vi "Phasor Explorer.vi"() -> ()   [LabVIEW 2019]
uses:
  Decay & Gates Options.ctl
  Phasor Explorer Phasor Plot Info.ctl
  SEPL Parameters.ctl
  Phasor Explorer Display Parameters.ctl
  Type of Series.ctl
  Phasor Explorer Phasor Parameters.ctl
  Phasor Calculation Type.ctl
  SEPL Type.ctl
  Phasor Explorer Decay Parameters.ctl
  IRF Model.ctl
  Phasor Explorer Gate Parameters.ctl
  Gate Type.ctl
  Type of User-defined Function.ctl
  Phasor Explorer Detector Parameters.ctl
  Phasor Explorer Q [Element].ctl
  Phasor Explorer Q [Event] List.ctl
  Phasor Explorer Internal Variables.ctl
  Graphs/XY Graph/XY Plot Data.ctl
  Graphs/XY Graph/XY Graph Plot Properties.ctl
  Graphs/XY Graph/XY Graph Event.ctl
  <vilib>/Utility/miscctls.llb/LVPoint32TypeDef.ctl
  <vilib>/Utility/miscctls.llb/LVPointDoubleTypeDef.ctl
  Graphs/Cursor Info.ctl
  SEPXP Globals.vi
  Phasor_Abort Parallel Computation.vi
  User-defined Gate.vi
  Graphs/Plot Editor/Plot Editor.lvlib
  Notebook/Notebook.lvlib
  Graphs/XY Graph/XY Graph Add-Ons.lvlib
  Rich Text Box/Rich Text Box.lvlib
  Variant/Variant to Data/Variant to Data.lvlib
panel:
  in  "Abort":bool
  in  "Message":string
  in  "Animated Busy Icon":bool=TRUE
  in  "Display Tabs":T1(tab)
  in  "Show UC Ticks":bool
  out "original tau_m":dbl[unit] format="%#_5g"
  out "original  tau_ph":dbl[unit] format="%#_5g"
  out "Phasor Graph TipStrip":string
  out "current tau_m":dbl[unit] format="%#_5g"
  out "current tau_ph":dbl[unit] format="%#_5g"
  out "tau_i":dbl[unit] format="%#_5g"
  out "Phasor Graph":cluster{"X Array":dbl[], "Y Array":dbl[]}[](graph)
  out "f(tau) Graph TipStrip":string
  out "Numerical Solution":T2 {"Solution 2" format="%#_5g"; "Solution 1" format="%#_5g"}
  out "Analytical Solutions":T2 caption="Analytical Solution" {"Solution 2" format="%#_5g"; "Solution 1" format="%#_5g"}
  in  "Use Cursor":bool caption="Use Pseudo Phasor Graph Cursor"
  in  "Linear Coefficients":cluster{"u":dbl, "v":dbl} {"v" format="%#_5g"; "u" format="%#_5g"}
  out "f(tau) Graph":cluster{"X Array":dbl[], "Y Array":dbl[]}[](graph)
  out "a(b) Graph TipStrip":string
  out "Max Tau":dbl[unit] format="%#_5g"
  out "Min Tau":dbl[unit] format="%#_5g"
  out "a(b) Graph":cluster{"X Array":dbl[], "Y Array":dbl[]}[](graph)=[{"X Array"=[0.0, 0.01, 0.02, 0.03, 0.04, 0.05, 0.060000000000000005, 0.07, 0.08, 0.09, 0.09999999999999999, 0.10999999999999999, 0.11999999999999998, 0.12999999999999998, 0.13999999999999999, 0.15, 0.16, 0.17, 0.18000000000000002, 0.19000000000000003, 0.20000000000000004, 0.21000000000000005, 0.22000000000000006, 0.23000000000000007, 0.24000000000000007, 0.25000000000000006, 0.26000000000000006, 0.2700000000000001, 0.2800000000000001, 0.2900000000000001, 0.3000000000000001, 0.3100000000000001, 0.3200000000000001, 0.3300000000000001, 0.34000000000000014, 0.35000000000000014, 0.36000000000000015, 0.37000000000000016, 0.38000000000000017, 0.3900000000000002, 0.4000000000000002, 0.4100000000000002, 0.4200000000000002, 0.4300000000000002, 0.4400000000000002, 0.45000000000000023, 0.46000000000000024, 0.47000000000000025, 0.48000000000000026, 0.49000000000000027, 0.5000000000000002, 0.5100000000000002, 0.5200000000000002, 0.5300000000000002, 0.5400000000000003, 0.5500000000000003, 0.5600000000000003, 0.5700000000000003, 0.5800000000000003, 0.5900000000000003, 0.6000000000000003, 0.6100000000000003, 0.6200000000000003, 0.6300000000000003, 0.6400000000000003, 0.6500000000000004, 0.6600000000000004, 0.6700000000000004, 0.6800000000000004, 0.6900000000000004, 0.7000000000000004, 0.7100000000000004, 0.7200000000000004, 0.7300000000000004, 0.7400000000000004, 0.7500000000000004, 0.7600000000000005, 0.7700000000000005, 0.7800000000000005, 0.7900000000000005, 0.8000000000000005, 0.8100000000000005, 0.8200000000000005, 0.8300000000000005, 0.8400000000000005, 0.8500000000000005, 0.8600000000000005, 0.8700000000000006, 0.8800000000000006, 0.8900000000000006, 0.9000000000000006, 0.9100000000000006, 0.9200000000000006, 0.9300000000000006, 0.9400000000000006, 0.9500000000000006, 0.9600000000000006, 0.9700000000000006, 0.9800000000000006, 0.9900000000000007, 1.0000000000000007], "Y Array"=[0.0, 0.01, 0.02, 0.03, 0.04, 0.05, 0.060000000000000005, 0.07, 0.08, 0.09, 0.09999999999999999, 0.10999999999999999, 0.11999999999999998, 0.12999999999999998, 0.13999999999999999, 0.15, 0.16, 0.17, 0.18000000000000002, 0.19000000000000003, 0.20000000000000004, 0.21000000000000005, 0.22000000000000006, 0.23000000000000007, 0.24000000000000007, 0.25000000000000006, 0.26000000000000006, 0.2700000000000001, 0.2800000000000001, 0.2900000000000001, 0.3000000000000001, 0.3100000000000001, 0.3200000000000001, 0.3300000000000001, 0.34000000000000014, 0.35000000000000014, 0.36000000000000015, 0.37000000000000016, 0.38000000000000017, 0.3900000000000002, 0.4000000000000002, 0.4100000000000002, 0.4200000000000002, 0.4300000000000002, 0.4400000000000002, 0.45000000000000023, 0.46000000000000024, 0.47000000000000025, 0.48000000000000026, 0.49000000000000027, 0.5000000000000002, 0.5100000000000002, 0.5200000000000002, 0.5300000000000002, 0.5400000000000003, 0.5500000000000003, 0.5600000000000003, 0.5700000000000003, 0.5800000000000003, 0.5900000000000003, 0.6000000000000003, 0.6100000000000003, 0.6200000000000003, 0.6300000000000003, 0.6400000000000003, 0.6500000000000004, 0.6600000000000004, 0.6700000000000004, 0.6800000000000004, 0.6900000000000004, 0.7000000000000004, 0.7100000000000004, 0.7200000000000004, 0.7300000000000004, 0.7400000000000004, 0.7500000000000004, 0.7600000000000005, 0.7700000000000005, 0.7800000000000005, 0.7900000000000005, 0.8000000000000005, 0.8100000000000005, 0.8200000000000005, 0.8300000000000005, 0.8400000000000005, 0.8500000000000005, 0.8600000000000005, 0.8700000000000006, 0.8800000000000006, 0.8900000000000006, 0.9000000000000006, 0.9100000000000006, 0.9200000000000006, 0.9300000000000006, 0.9400000000000006, 0.9500000000000006, 0.9600000000000006, 0.9700000000000006, 0.9800000000000006, 0.9900000000000007, 1.0000000000000007]}]
  in  "Compute Delta Tau":bool
  out "Pseudo-Phase Lifetime Graph TipStrip":string
  out "Pseudo-Phase Lifetime Graph":cluster{"X Array":dbl[], "Y Array":dbl[]}[](graph)=[{"X Array"=[0.0, 1.0, 2.0, 3.0, 4.0, 5.0, 6.0, 7.0, 8.0, 9.0, 10.0, 11.0, 12.0, 13.0, 14.0, 15.0, 16.0, 17.0, 18.0, 19.0, 20.0, 21.0, 22.0, 23.0, 24.0, 25.0, 26.0, 27.0, 28.0, 29.0, 30.0, 31.0, 32.0, 33.0, 34.0, 35.0, 36.0, 37.0, 38.0, 39.0, 40.0, 41.0, 42.0, 43.0, 44.0, 45.0, 46.0, 47.0, 48.0, 49.0, 50.0, 51.0, 52.0, 53.0, 54.0, 55.0, 56.0, 57.0, 58.0, 59.0, 60.0, 61.0, 62.0, 63.0, 64.0, 65.0, 66.0, 67.0, 68.0, 69.0, 70.0, 71.0, 72.0, 73.0, 74.0, 75.0, 76.0, 77.0, 78.0, 79.0, 80.0, 81.0, 82.0, 83.0, 84.0, 85.0, 86.0, 87.0, 88.0, 89.0, 90.0, 91.0, 92.0, 93.0, 94.0, 95.0, 96.0, 97.0, 98.0, 99.0, 100.0], "Y Array"=[0.0, 1.0, 2.0, 3.0, 4.0, 5.0, 6.0, 7.0, 8.0, 9.0, 10.0, 11.0, 12.0, 13.0, 14.0, 15.0, 16.0, 17.0, 18.0, 19.0, 20.0, 21.0, 22.0, 23.0, 24.0, 25.0, 26.0, 27.0, 28.0, 29.0, 30.0, 31.0, 32.0, 33.0, 34.0, 35.0, 36.0, 37.0, 38.0, 39.0, 40.0, 41.0, 42.0, 43.0, 44.0, 45.0, 46.0, 47.0, 48.0, 49.0, 50.0, 51.0, 52.0, 53.0, 54.0, 55.0, 56.0, 57.0, 58.0, 59.0, 60.0, 61.0, 62.0, 63.0, 64.0, 65.0, 66.0, 67.0, 68.0, 69.0, 70.0, 71.0, 72.0, 73.0, 74.0, 75.0, 76.0, 77.0, 78.0, 79.0, 80.0, 81.0, 82.0, 83.0, 84.0, 85.0, 86.0, 87.0, 88.0, 89.0, 90.0, 91.0, 92.0, 93.0, 94.0, 95.0, 96.0, 97.0, 98.0, 99.0, 100.0]}]
  out "Decay & Gates Graph TipStrip":string
  in  "Decay & Gates Options":T3
  out "Decay & Gates Graph":cluster{"X Array":dbl[], "Y Array":dbl[]}[](graph)
  in  "Version":enum32{"Version 1", "Version 2"}(radio)=enum."Version 2"
  out "Sum of Gates Graph TipStrip":string
  out "Sum of Gates Graph":cluster{"X Array":dbl[], "Y Array":dbl[]}[](graph)
  out "Phasor Graph Plots Metadata":T4[](array[typedef]) {"Phasor Explorer Parameters"."Detector Parameters"."Frames/Image" min=1; "Phasor Explorer Parameters"."Detector Parameters"."Multiplicity" min=0; "Phasor Explorer Parameters"."Detector Parameters"."Bits/Frame" min=1; "Phasor Explorer Parameters"."Detector Parameters"."Gates/Frame" min=1; "Phasor Explorer Parameters"."Gate Parameters"."# Steps" min=0.0; "Phasor Explorer Parameters"."Gate Parameters"."Tolerance" min=0.0; "Phasor Explorer Parameters"."Gate Parameters"."Top Slope" min=0.0; "Phasor Explorer Parameters"."Gate Parameters"."Edge Width" min=0.0; "Phasor Explorer Parameters"."Gate Parameters"."Gate Step" min=0.0; "Phasor Explorer Parameters"."Gate Parameters"."# Gates" min=0.0 step=1.0; "Phasor Explorer Parameters"."Gate Parameters"."Gate Width" min=0.0; "Phasor Explorer Parameters"."Decay & IRF Parameters"."Lifetime" min=0.0; "Phasor Explorer Parameters"."Decay & IRF Parameters"."IRF Period" min=0.0; "Phasor Explorer Parameters"."Phasor Parameters"."Square Gate Width" min=0.0; "Phasor Explorer Parameters"."Phasor Parameters"."# Gates" min=0.0; "Phasor Explorer Parameters"."Phasor Parameters"."Calibration Lifetime" min=0.0; "Phasor Explorer Parameters"."Phasor Parameters"."Harmonic Frequency" min=0.0; "Phasor Explorer Parameters"."Display Parameters"."Min tau" min=0.0; "Phasor Explorer Parameters"."Display Parameters"."Max tau" min=0.0; "Phasor Explorer Parameters"."Display Parameters"."# Points" min=1 step=1}
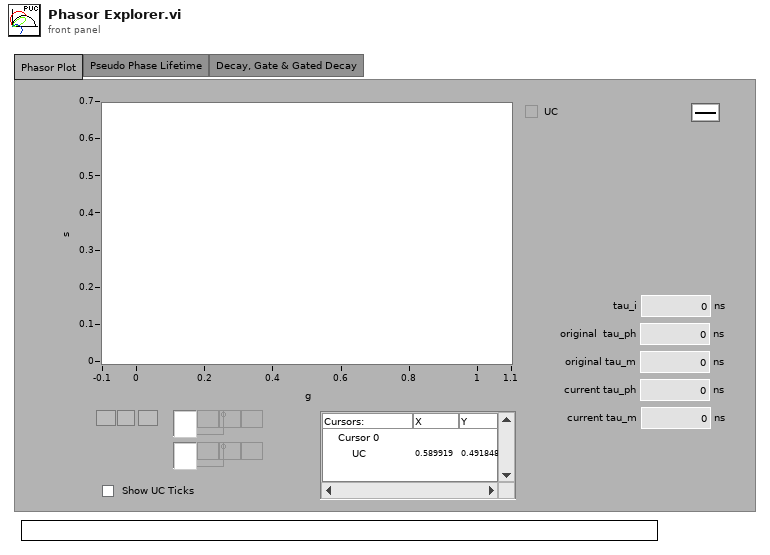
[diagram p1: front panel]
types:
  T1 = enum32{"Phasor Plot", "UC Intersections", "Alpha vs Beta", "Pseudo Phase Lifetime", "Decay, Gate & Gated Decay", "Sum of Gates", "Debug"}
  T2 = cluster{"Solution 1":dbl[unit], "Solution 2":dbl[unit]}
  T3 = typedef "Decay & Gates Options.ctl" = cluster{"Decay":bool, "Gate":bool, "Gated Decay":bool}
  T4 = typedef "Phasor Explorer Phasor Plot Info.ctl" = cluster{"Lifetime/Fraction Array":dbl[], "Phasor Explorer Parameters":T5, "Phase Lifetimes":dbl[], "Modulus Lifetimes":dbl[]}
  T5 = typedef "SEPL Parameters.ctl" = cluster{"Display Parameters":T6, "Phasor Parameters":T8, "Decay & IRF Parameters":T11, "Gate Parameters":T13, "Detector Parameters":T16}
  T6 = typedef "Phasor Explorer Display Parameters.ctl" = cluster{"# Points":i32, "Ramp Type":enum16{"Linear", "Logarithmic"}, "Type of Series":T7, "Min tau":dbl[unit], "Max tau":dbl[unit], "Include 0":bool, "Include Infinity":bool}
  T7 = typedef "Type of Series.ctl" = enum16{"1-Exp Decays", "Linear Combination of 1-Exp"}
  T8 = typedef "Phasor Explorer Phasor Parameters.ctl" = cluster{"Harmonic Frequency":dbl[unit], "Use f* = 1/D Frequency":bool, "Calibrated Phasor":bool, "Calibration Lifetime":dbl[unit], "Phasor Calculation":T9, "SEPL Type":T10, "# Gates":dbl, "Square Gate Width":dbl[unit], "Show Ticks":bool}
  T9 = typedef "Phasor Calculation Type.ctl" = enum16{"Direct Sum", "Analytical Formula"}
  T10 = typedef "SEPL Type.ctl" = enum16{"UC", "L_N", "L_N[W]", "L_X"}
  T11 = typedef "Phasor Explorer Decay Parameters.ctl" = cluster{"Lifetime":dbl[unit], "IRF Offset":dbl[unit], "IRF Period":dbl[unit], "Normalized Decays":bool, "IRF Model":T12, "IRF Parameter 1":dbl[unit]}
  T12 = typedef "IRF Model.ctl" = enum16{"Dirac", "Exponential"}
  T13 = typedef "Phasor Explorer Gate Parameters.ctl" = cluster{"First Gate Start":dbl[unit], "Use Gate Center":bool, "Gate Width":dbl[unit], "Gate Step":dbl[unit], "# Gates":dbl, "Gate Type":T14, "Edge Width":dbl[unit], "Top Slope":dbl[unit], "Reversed Sawtooth?":bool, "Analytical Computation":bool, "Integration":enum32{"Item 0", "Item 1"}, "Tolerance":dbl, "# Steps":dbl, "Type of User-defined Function":T15, "Use Gate Step":bool}
  T14 = typedef "Gate Type.ctl" = enum16{"Square", "Finite Edge Square", "Finite Edge, Tilted Top Square", "Triangle", "Sawtooth", "User-defined"}
  T15 = typedef "Type of User-defined Function.ctl" = enum16{"Gate", "IRF"}
  T16 = typedef "Phasor Explorer Detector Parameters.ctl" = cluster{"Frames/Image":i32, "Gates/Frame":i32, "Bits/Frame":i32, "Multiplicity":i32, "Incident Signal":dbl, "Poisson Signal":bool}
  T17 = typedef "Phasor Explorer Q [Event] List.ctl" = enum16{"Idle", "Initialization", "Show-Hide UC Ticks", "Edit User-defined Gate/IRF", "Update Phasor Graph", "Update Sum of Gates Graph", "Update Parameters", "Compute Decay &/or Gates", "Find Pseudo UC Intersections", "Compute alpha(beta) Plot", "Compute Pseudo-Phase Lifetime Plot", "Export Parameters to Clipboard", "Update Phase & Modulus Lifetime", "XY Graph Special Event", "Update Graph Plots Info", "Fit to Circle", "Quit"}
  T18 = enum32{"Phasor Plot", "UC Intersections", "Alpha vs Beta", "Pseudo Phase Lifetime", "Decay, Gate & Gated Decay", "Sum of Gates", "Debug"}[]
  T19 = typedef "Phasor Explorer Internal Variables.ctl" = cluster{"User-Defined Gate":T20, "User-defined Gate Plot Style":T21, "User-Defined IRF":T20}
  T20 = typedef "XY Plot Data.ctl" = cluster{"X Array":dbl[], "Y Array":dbl[]}
  T21 = typedef "XY Graph Plot Properties.ctl" = cluster{"Plot Index":i32, "Plot.Bar Plot Style":u8, "Plot.DigitalLineStyle":u8, "Plot.TransitionLocation":u8, "Plot.Transition Type":u8, "Plot.Fill To":i16, "Plot.Fill/Pt. Color":u32, "Plot.Label Format":u8, "Plot.Line Style":u8, "Plot.Line Width":u8, "Plot.Plot Color":u32, "Plot.Plot Interpolation":u8, "Plot.Plot Name":string, "Plot.Point Style":u8, "Plot.Visible?":bool, "Plot.XScaleIdx":u32, "Plot.YScaleIdx":u32, "Plot.Anti-aliased":bool}
  T22 = typedef "Phasor Explorer Q [Element].ctl" = cluster{"ZXP Q Event":T17, "Data":variant}
  T23 = typedef "Phasor Explorer Tipstrip Event Registration Refnums.ctl" = cluster{"Phasor Graph Event Registration Refnum":refnum<event-registration>, "Sum of Gates Graph Event Registration Refnum":refnum<event-registration>, "f(tau) Graph Event Registration Refnum":refnum<event-registration>, "a(b) Graph Event Registration Refnum":refnum<event-registration>, "Pseudo-Phase Lifetime Graph Event Registration Refnum":refnum<event-registration>, "Decay & Gate Graph Event Registration Refnum":refnum<event-registration>}
  T24 = enum32{"Phasor Plot", "UC Intersections", "Alpha vs Beta", "Pseudo Phase Lifetime", "Decay, Gate & Gated Decay", "Sum of Gates"}
  T25 = typedef "Cursor Info.ctl" = cluster{"CtlRef":refnum<vi>, "CursIdx":i32, "CursRef":refnum<vi>, "PlotIdx":i32, "PointIdx":i32, "CursLoc":cluster{"X":dbl, "Y":dbl}}
  T26 = typedef "XY Graph Add-Ons.lvlib/XY Graph Event.ctl" = cluster{"Item Tag":string, "XY Graph Refnum":refnum<vi>, "Coords":T27, "Item Path":string}
  T27 = typedef "LVPoint32TypeDef.ctl" = cluster{"Horizontal":i32, "Vertical":i32}
  T28 = typedef "LVPointDoubleTypeDef.ctl" = cluster{"X":dbl, "Y":dbl}
  T29 = cluster{"XY Graph Ref":refnum<vi>, "Mouse Coordinates":T28, "Plot Index":i32}
  T30 = typedef "Rich Text Box.lvlib/Text Formatting.ctl" = cluster{"Font":string, "Text Color":T31, "Text Background Color":T31, "Text Style":enum16{"Regular", "Bold", "Italic", "Underline", "Strikeout"}, "Font Size (Points)":dbl, "Text Alignment":i32}
  T31 = typedef "Rich Text Box.lvlib/Text Colors.ctl" = enum16{"Unchanged", "Black", "Blue", "Brown", "Gray", "Green", "Orange", "Pink", "Red", "White"}
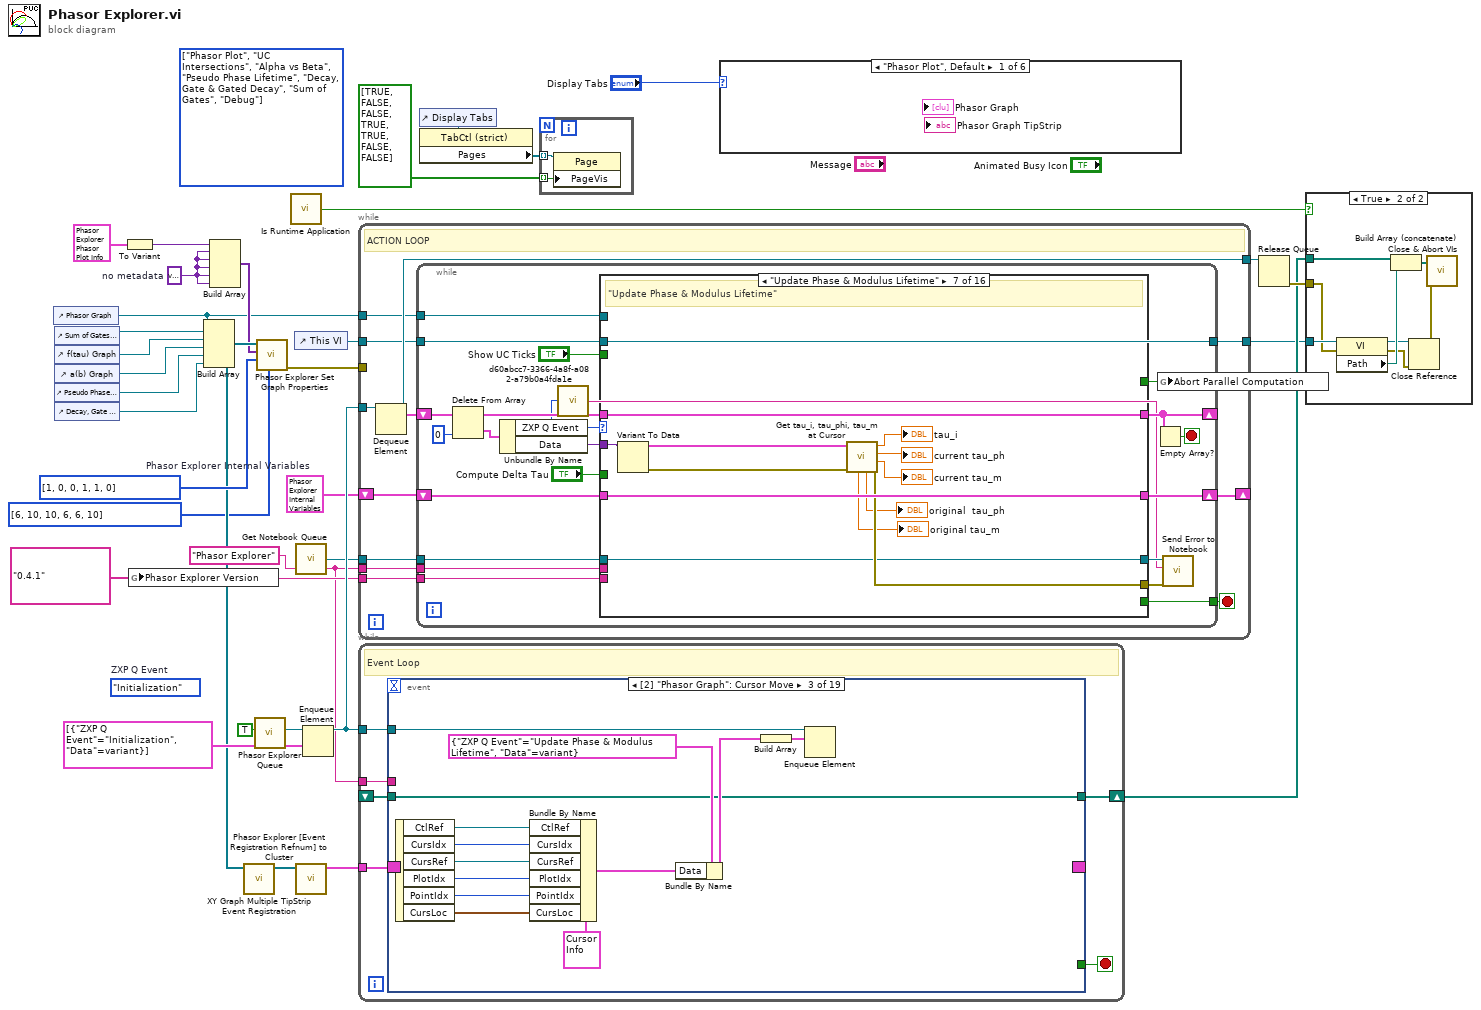
[diagram p0: block diagram]
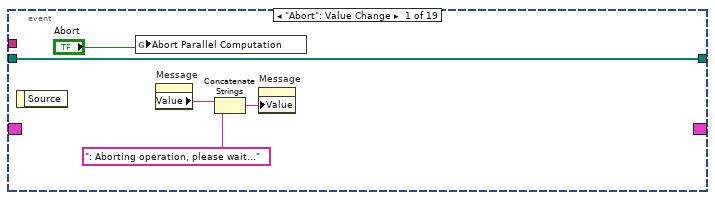
[diagram p3: hidden frame]
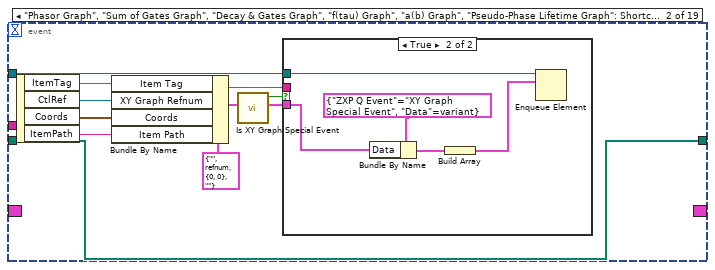
[diagram p4: hidden frame]
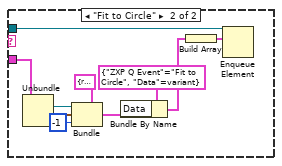
[diagram p6: hidden frame]
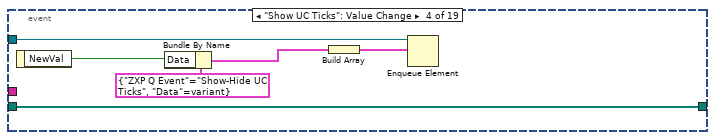
[diagram p7: hidden frame]
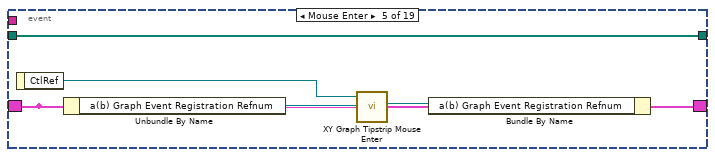
[diagram p8: hidden frame]
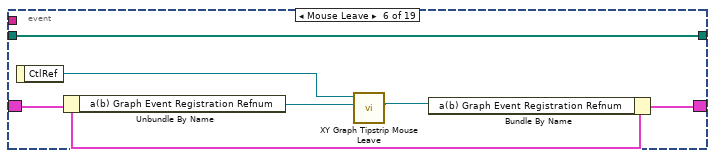
[diagram p9: hidden frame]
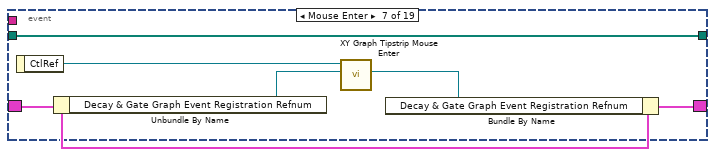
[diagram p10: hidden frame]
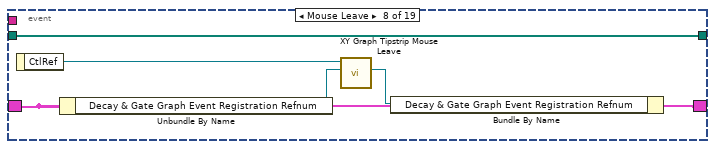
[diagram p11: hidden frame]
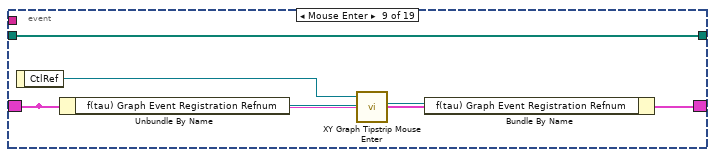
[diagram p12: hidden frame]
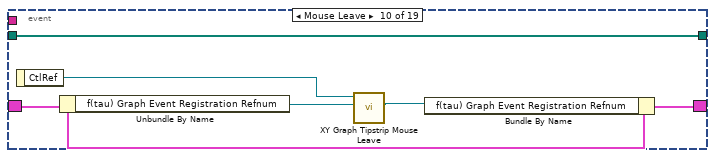
[diagram p13: hidden frame]
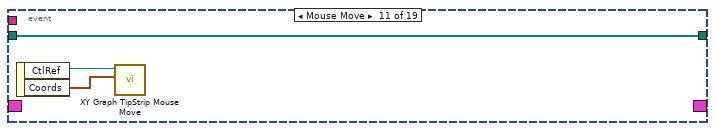
[diagram p14: hidden frame]
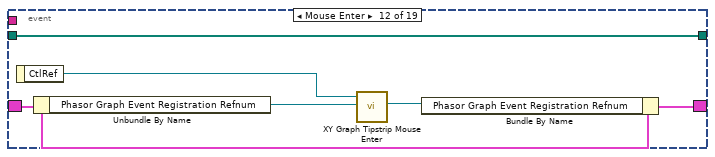
[diagram p15: hidden frame]
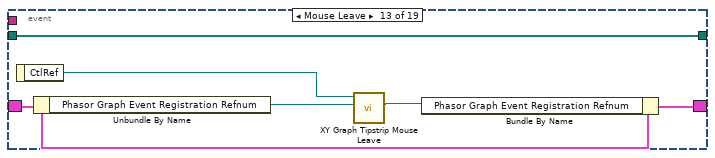
[diagram p16: hidden frame]
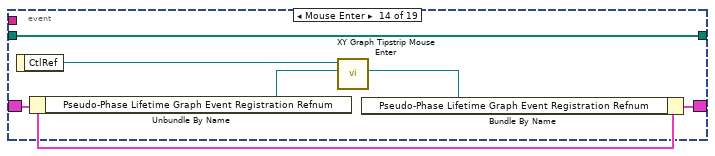
[diagram p17: hidden frame]
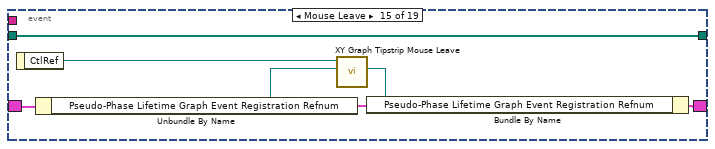
[diagram p18: hidden frame]
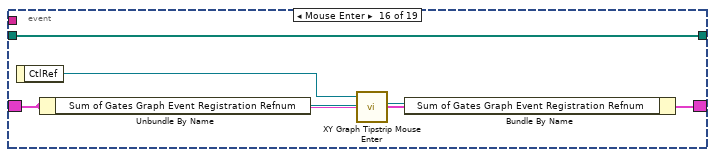
[diagram p19: hidden frame]
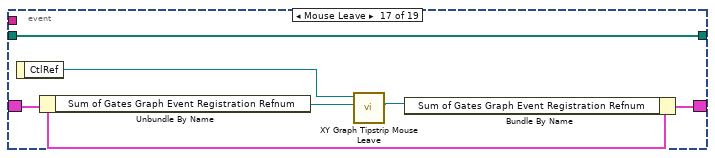
[diagram p20: hidden frame]
diagram:
  (unwired) Phasor_Explorer_Q_[Event]_List."Initialization"  # ZXP Q Event
  (unwired) T18 [enum."Phasor Plot", enum."UC Intersections", enum."Alpha vs Beta", enum."Pseudo Phase Lifetime", enum."Decay, Gate & Gated Decay", enum."Sum of Gates", enum."Debug"] items=["Phasor Plot", "UC Intersections", "Alpha vs Beta", "Pseudo Phase Lifetime", "Decay, Gate & Gated Decay", "Sum of Gates", "Debug"] ("Display Tabs")
  w9 = variant  # no metadata
  w15 = "Phasor Explorer" ("Phasor Explorer Version")
  w28 = "0.4.1" ("Phasor Explorer Version")
  w31 = T19 {"User-Defined Gate"={"X Array"=[], "Y Array"=[]}, "User-defined Gate Plot Style"={"Plot Index"=0, "Plot.Bar Plot Style"=0, "Plot.DigitalLineStyle"=0, "Plot.TransitionLocation"=0, "Plot.Transition Type"=0, "Plot.Fill To"=-1, "Plot.Fill/Pt. Color"=0, "Plot.Label Format"=0, "Plot.Line Style"=0, "Plot.Line Width"=0, "Plot.Plot Color"=0, "Plot.Plot Interpolation"=4, "Plot.Plot Name"="User-defined Gate", "Plot.Point Style"=0, "Plot.Visible?"=TRUE, "Plot.XScaleIdx"=0, "Plot.YScaleIdx"=0, "Plot.Anti-aliased"=TRUE}, "User-Defined IRF"={"X Array"=[], "Y Array"=[]}}  # Phasor Explorer Internal Variables
  n1 = control-ref of="Phasor Graph"() -> (w8:refnum<vi>)
  n2 = control-ref of="Sum of Gates Graph"() -> (w26:refnum<vi>)
  n3 = control-ref of="f(tau) Graph"() -> (w25:refnum<vi>)
  n4 = control-ref of="a(b) Graph"() -> (w24:refnum<vi>)
  n5 = control-ref of="Pseudo Phase Lifetime Graph"() -> (w23:refnum<vi>)
  n6 = control-ref of="Decay, Gate & Gated Decay Graph"() -> (w22:refnum<vi>)
  n7 = To Variant(anything=T4 {"Lifetime/Fraction Array"=[], "Phasor Explorer Parameters"={"Display Parameters"={"# Points"=0, "Ramp Type"=enum."Linear", "Type of Series"=enum."1-Exp Decays", "Min tau"=0.0, "Max tau"=0.0, "Include 0"=FALSE, "Include Infinity"=FALSE}, "Phasor Parameters"={"Harmonic Frequency"=0.0, "Use f* = 1/D Frequency"=FALSE, "Calibrated Phasor"=FALSE, "Calibration Lifetime"=1e-09, "Phasor Calculation"=enum."Direct Sum", "SEPL Type"=enum."UC", "# Gates"=1.0, "Square Gate Width"=1e-09, "Show Ticks"=FALSE}, "Decay & IRF Parameters"={"Lifetime"=0.0, "IRF Offset"=0.0, "IRF Period"=0.0, "Normalized Decays"=FALSE, "IRF Model"=enum."Dirac", "IRF Parameter 1"=0.0}, "Gate Parameters"={"First Gate Start"=0.0, "Use Gate Center"=FALSE, "Gate Width"=0.0, "Gate Step"=0.0, "# Gates"=0.0, "Gate Type"=enum."Square", "Edge Width"=0.0, "Top Slope"=0.0, "Reversed Sawtooth?"=FALSE, "Analytical Computation"=FALSE, "Integration"=enum."Item 0", "Tolerance"=1.0, "# Steps"=1.0, "Type of User-defined Function"=enum."Gate", "Use Gate Step"=FALSE}, "Detector Parameters"={"Frames/Image"=0, "Gates/Frame"=0, "Bits/Frame"=0, "Multiplicity"=0, "Incident Signal"=0.0, "Poisson Signal"=FALSE}}, "Phase Lifetimes"=[], "Modulus Lifetimes"=[]} ("Phasor Graph Plot Info")) -> (Variant=w11:variant)
  n8 = global write "SEPXP Globals.vi" "Phasor Explorer Version"(w28) -> ()
  n9 = Build Array(w8, w26, w25, w24, w23, w22) -> (w19:refnum<vi>[])
  n10 = Build Array(w11, w9, w9, w9, w9, w9) -> (w10:variant[])
  n11 = call "XY Graph Multiple TipStrip Event Registration.vi"("XY Graph Refnums"=w19) -> ("Tipstrips Event Registrations"=w18:refnum<event-registration>[])  [unwired: 9 in, 1 out]
  n12 = call "Phasor Explorer Queue.vi"("create if not found? (F)"=TRUE) -> ("Phasor Explorer Queue"=w14:refnum<queue>)  [unwired: 10 in]
  n13 = call "Phasor Explorer Set Graph Properties.vi"("Max Legend Size (8)"=i32[] [6, 10, 10, 6, 6, 10], "# Preserved PLots"=i32[] [1, 0, 0, 1, 1, 0], "Metadata Type"=w10, "XY Graph Ref Array"=w19) -> ("Error Out"=w21:errorcluster)  [unwired: 7 in]
  n14 = call "Is Runtime Application.vi"() -> ("Runtime ?"=w2:bool)  [unwired: 8 in, 1 out]
  n15 = control-ref of="This VI"() -> (w7:refnum<vi>)
  n16 = call "Get Notebook Queue.vi"() -> ("Notebook Queue"=w29:refnum<queue>)  [unwired: 9 in]
  n17 = call "Phasor Explorer [Event Registration Refnum] to Cluster.vi"("Tipstrips Event Registrations"=w18) -> ("Tipstrip RE refnums"=w17:T23)  [unwired: 10 in]
  n18 = Enqueue Element(queue=w14, element=T22[] [{"ZXP Q Event"=enum."Initialization", "Data"=variant}] ("PSEXP Q Element")) -> (queue out=w32:refnum<queue>)  [unwired: 2 in, 2 out]
  n19 = while {
    tunnel: w32 -> [w46]
    tunnel: [w44] -> w33
    tunnel: w7 -> [w42]
    shift-right: [w40] -> _
    shift-left: w31 -> [w41]
    tunnel: w29 -> [w39]
    tunnel: w28 -> [w38]
    tunnel: w15 -> [w37]
    tunnel: w21 -> [_]
    tunnel: w8 -> [w36]
    tunnel: [w35] -> w1
    stop <- w43 stop-if-true
    # "ACTION LOOP"
    n20 = Dequeue Element(queue=w46) -> (queue out=w44:refnum<queue>, element=w45:T22[])  [unwired: 2 in, 2 out]
    n21 = while {
      shift-right: [w64] -> _
      shift-left: w45 -> [w66]
      tunnel: [w62] -> w43
      tunnel: w42 -> [w48]
      shift-right: [w60] -> w40
      shift-left: w41 -> [w61]
      tunnel: w39 -> [w58]
      tunnel: w38 -> [w57]
      tunnel: w37 -> [w56]
      tunnel: w36 -> [w50]
      tunnel: [w48] -> w35
      stop <- w63 stop-if-true
      n22 = Delete From Array(array=w66, index=0) -> (deleted portion=w67:T22, array with subset deleted=w65:T22[])  [unwired: 1 in]
      n23 = Unbundle By Name(w67) -> ("ZXP Q Event"=w52:T17, "Data"=w59:variant)
      n24 = call "d60abcc7-3366-4a8f-a082-a79b0a4fda1e.vi"("Enum"=w52) -> ("String"=w51:string)
      n25 = case shown="\"Update Phase & Modulus Lifetime\"" w52 {
        tunnel: w65 -> [w71 w93 w122 w139 w160 w168 w180 w192 w201 w207 w217 w239 w248 w255 w266 _]
        tunnel: [w71 w93 w122 w139 w160 w168 w180 w192 w201 w207 w217 w239 w248 w255 w266 T22[] []] -> w64
        tunnel: [_ _ _ _ _ _ _ _ _ _ _ _ _ _ _ w271] -> w62
        tunnel: w48 -> [_ _ _ _ w157 w164 _ w183 w196 _ w211 w235 _ _ _ _]
        tunnel: w61 -> [w70 w77 w120 w126 w152 w165 w174 w189 w198 w204 w212 w236 w247 w254 w265 w275]
        tunnel: [w70 w77 w120 w127 w152 w165 w174 w189 w198 w204 w212 w236 w247 w254 w265 w275] -> w60
        tunnel: w59 -> [_ _ w109 w135 _ _ w179 _ _ _ _ _ w244 _ w264 _]
        tunnel: w58 -> [w69 w84 w121 w136 w153 w161 w172 w181 w193 w202 w208 w218 w240 w253 w261 w272]
        tunnel: w57 -> [_ w92 _ _ _ _ _ _ _ _ _ _ _ _ _ w274]
        tunnel: w56 -> [_ w91 _ _ _ _ _ _ _ _ _ _ _ _ _ w268]
        tunnel: "Compute Delta Tau" -> [_ _ _ _ _ _ _ _ w195 _ _ _ _ _ _ _]
        tunnel: [_ w86 w113 w137 w154 w162 w173 w182 w194 w203 w209 w219 w241 _ w259 w270] -> w54
        tunnel: [w69 w84 w121 w136 w153 w161 w172 w181 w193 w202 w208 w218 w240 w253 w261 w272] -> w53
        tunnel: w50 -> [_ w82 w115 _ _ _ _ _ _ _ _ _ _ w252 _ _]
        tunnel: [_ _ _ _ FALSE ("Abort") _ _ _ _ _ _ _ _ _ _ _] -> w47
        tunnel: "Show UC Ticks" -> [_ w72 _ _ _ _ _ _ _ _ _ _ _ _ _ _]
        frame "Idle", Default {
          # "\"Idle\", Default"
        }
        frame "Initialization" {
          # "\"Initialization\""
          n26 = call "Send Start-Stop Message.vi"("Start(T)/Stop(F)"=TRUE, "Version number"=w92, "Software Name"=w91, "Notebook Queue"=w84) -> ("Error Out"=w85:errorcluster)  [unwired: 7 in]
          n27 = call "Phasor Explorer Save-Load Settings.vi"("Load(F)/Save (T)"=FALSE) -> ("Error Out"=w89:errorcluster)  [unwired: 9 in, 1 out]
          n28 = call "9d87ee79-5232-47ce-8c93-ac6730099a75.vi"("# Steps (1)"=100) -> ("Ramp"=w101:dbl[])  [unwired: 8 in, 2 out]
          n29 = call "79f5c63b-0c71-4b9b-95d4-cbcc2b15c9cb.vi"("# Steps (1)"=100, "End (1)"=100.0) -> ("Ramp"=w106:dbl[])  [unwired: 7 in, 2 out]
          n30 = call "Get Harmonic Frequency.vi"("Error In"=w89) -> ("Error Out"=w75:errorcluster, "Harmonic frequency"=w76:dbl[unit])  [unwired: 2 in, 1 out]
          n31 = Bundle("Ramp"=w101, "Ramp"=w101) -> (w103:cluster{"Ramp":dbl[], "Ramp":dbl[]})  [unwired: 1 in]
          n32 = Bundle("Ramp"=w106, "Ramp"=w106) -> (w104:cluster{"Ramp":dbl[], "Ramp":dbl[]})  [unwired: 1 in]
          n33 = call "Universal Semicircle Plot.vi"("Error In"=w75, "Show Ticks"=w72, "Harmonic frequency"=w76) -> ("Error Out"=w74:errorcluster, "Universal Semi-circle"=w80:cluster{"X Array":dbl[], "Y Array":dbl[]})  [unwired: 6 in, 1 out]
          n34 = Build Array(w103) -> (w102:cluster{"Ramp":dbl[], "Ramp":dbl[]}[])
          n35 = Build Array(w104) -> (w105:cluster{"Ramp":dbl[], "Ramp":dbl[]}[])
          n36 = call "Phasor Explorer Update UC Lifetimes.vi"("Error In"=w74, "Harmonic Frequency"=w76, "Universal Semi-circle"=w80) -> ("Error Out"=w73:errorcluster, "PhXP UC Plot Info out"=w81:T4)  [unwired: 7 in]
          n37 = property on="a(b) Graph" class="XYGraph (strict)"("Value"=w102, "Active Plot"=u32 0, "Plot.Plot Name"="alpha = beta") -> ()  [unwired: 2 in, 2 out]
          n38 = property on="Pseudo-Phase Lifetime Graph" class="XYGraph (strict)"("Value"=w105, "Active Plot"=u32 0, "Plot.Plot Name"="tau = P-tau_ph") -> ()  [unwired: 2 in, 2 out]
          n39 = call "XY Graph Add Single Plot with Name.vi"("XYGraph Ref in"=w82, "Keep Existing Plots (T)"=FALSE, "Plot"=w80, "Plot Metadata"=w81, "Plot Name (\"Plot\")"="UC" ("Plot.Plot Name"), "error in (no error)"=w73) -> ("error out"=w78:errorcluster)  [unwired: 6 in, 3 out]
          n40 = Merge Errors(w78, w85) -> (w86:errorcluster)
          n41 = local write "Display Tabs"(T24."Phasor Plot" ("Display Tabs")) -> ()
        }
        frame "Show-Hide UC Ticks" {
          w112 = 0 ("Plot Idx")
          # "\"Show-Hide UC Ticks\""
          n42 = call "Variant to Boolean.vi"("Variant"=w109) -> ("Value"=w108:bool)  [unwired: 8 in]
          n43 = call "Get Harmonic Frequency.vi"() -> ("Error Out"=w119:errorcluster, "Harmonic frequency"=w118:dbl[unit])  [unwired: 3 in, 1 out]
          n44 = call "Universal Semicircle Plot.vi"("Tick Length"=0.02, "Error In"=w119, "Show Ticks"=w108, "Harmonic frequency"=w118) -> ("Error Out"=w117:errorcluster, "Universal Semi-circle"=w110:cluster{"X Array":dbl[], "Y Array":dbl[]})  [unwired: 5 in, 1 out]
          n45 = call "Phasor Explorer Update UC Lifetimes.vi"("Error In"=w117, "Harmonic Frequency"=w118, "Universal Semi-circle"=w110) -> ("Error Out"=w116:errorcluster, "PhXP UC Plot Info out"=w111:T4)  [unwired: 7 in]
          n46 = call "XY Graph Update Plot.vi"("Error In"=w116, "Plot"=w110, "Plot Idx"=w112, "XY Graph refnum"=w115) -> ("Error Out"=w114:errorcluster)  [unwired: 7 in]
          n47 = call "XY Graph Set Plot Metdata.vi"("error in (no error)"=w114, "Plot Metadata"=w111, "Plot Index (-1: last)"=w112, "XYGraph Ref in"=w115) -> ("error out"=w113:errorcluster)  [unwired: 5 in, 2 out]
        }
        frame "Edit User-defined Gate/IRF" {
          w125 = Type_of_User-defined_Function."IRF" ("Type of User-defined Function")
          # "\"Edit User-defined Gate/IRF\""
          n48 = Unbundle By Name(w126) -> ("User-Defined IRF"=w130:T20, "User-Defined Gate"=w131:T20, "User-defined Gate Plot Style"=w138:T21)
          n49 = Variant To Data(type=w125, Variant=w135) -> (data=w124:T15)  [unwired: 1 in, 1 out]
          n50 = Equal?(x=w125, y=w124) -> (x = y?=w123:bool)
          n51 = Select(t=w130, s=w123, f=w131) -> (s? t:f=w129:T20)
          n52 = Format Into String(format string="User-Defined %s Plot" ("Original Graph Name"), w124) -> (resulting string=w133:string)  [unwired: 2 in, 1 out]
          n53 = call "Plot Editor.vi"("Original Graph Name"=w133, "Plot Style in"=w138, "Plot in"=w129) -> ("Error Out"=w137:errorcluster, "Plot Style out"=w128:T21, "Plot out"=w132:T20)  [unwired: 6 in]
          n54 = case shown="\"Gate\", Default" w124 {
            tunnel: w132 -> [w140 w144]
            tunnel: w128 -> [w143 w147]
            tunnel: [w142 w146] -> w127
            tunnel: w126 -> [w141 w145]
            frame "Gate", Default {
              n55 = Bundle By Name(cluster=w141, "User-Defined Gate"=w140, "User-defined Gate Plot Style"=w143) -> (w142:T19)
              n56 = global write "User-defined Gate.vi" "User-defined Gate"(w140) -> ()
            }
            frame "IRF" {
              n57 = Bundle By Name(cluster=w145, "User-Defined IRF"=w144, "User-defined Gate Plot Style"=w147) -> (w146:T19)
              n58 = global write "User-defined Gate.vi" "User-defined IRF"(w144) -> ()
            }
          }
        }
        frame "Update Phasor Graph" {
          # "\"Update Phasor Graph\""
          n59 = call "Show Animated Busy Icon with Message and Abort Button.vi"("Message"="Computing Phasor Graph...") -> ("Error Out"=w159:errorcluster)  [unwired: 18 in]
          n60 = call "Compute SEPL Wrapper.vi"("error in (no error)"=w159, "VI in"=w157) -> ("error out"=w158:errorcluster, "Notebook String"=w149:string, "Plot Name"=w150:string)  [unwired: 7 in]
          n61 = call "Hide Animated Busy Icon with Message and Abort Button.vi"("Error In"=w158) -> ("Error Out"=w151:errorcluster)  [unwired: 18 in]
          n62 = call "Send PhXP Phasor Plot Info to Notebook.vi"("Graph Type"="Phasor", "error in (no error)"=w151, "Phasor Plot Info String"=w149, "Plot Name"=w150, "Notebook Queue"=w153) -> ("Error Out"=w154:errorcluster)  [unwired: 6 in]
        }
        frame "Update Sum of Gates Graph" {
          # "\"Update Sum of Gates Graph\""
          n63 = call "Show Animated Busy Icon with Message and Abort Button.vi"("Message"="Computing Sum of Gates...", "Target VI reference"=w164) -> ("Error Out"=w167:errorcluster)  [unwired: 17 in]
          n64 = call "Compute Sum of Gates Plot Wrapper.vi"("error in (no error)"=w167, "VI in"=w164) -> ("error out"=w166:errorcluster)  [unwired: 9 in]
          n65 = call "Hide Animated Busy Icon with Message and Abort Button.vi"("Error In"=w166) -> ("Error Out"=w162:errorcluster)  [unwired: 18 in]
        }
        frame "Update Phase & Modulus Lifetime" {
          # "\"Update Phase & Modulus Lifetime\""
          n66 = Variant To Data(Variant=w179) -> (data=w169:T25, error out=w175:errorcluster)  [unwired: 2 in]
          n67 = call "Get tau_i, tau_phi, tau_m at Cursor.vi"("Error In"=w175, "Cursor Info"=w169) -> ("Error Out"=w173:errorcluster, "current tau_m"=→"current tau_m":dbl[unit], "current tau_ph"=→"current tau_ph":dbl[unit], "tau_i"=→"tau_i":dbl[unit], "original tau_ph"=→"original  tau_ph":dbl[unit], "original tau_m"=→"original tau_m":dbl[unit])  [unwired: 4 in]
        }
        frame "Compute Decay &/or Gates" {
          # "\"Compute Decay &/or Gates\""
          n68 = call "Show Animated Busy Icon with Message and Abort Button.vi"("Message"="Computing Decay/Gates...", "Target VI reference"=w183) -> ("Error Out"=w191:errorcluster)  [unwired: 17 in]
          n69 = call "Compute Decay & Time Gates Wrapper.vi"("error in (no error)"=w191, "VI in"=w183) -> ("error out"=w190:errorcluster, "Decay & Gates Plot String"=w187:string, "Added Plot Name(s)"=w184:string)  [unwired: 6 in, 1 out]
          n70 = call "Hide Animated Busy Icon with Message and Abort Button.vi"("Target VI reference"=w183, "Error In"=w190) -> ("Error Out"=w186:errorcluster)  [unwired: 17 in]
          n71 = call "Send PhXP Phasor Plot Info to Notebook.vi"("Graph Type"="Decay & Gates", "error in (no error)"=w186, "Phasor Plot Info String"=w187, "Plot Name"=w184, "Notebook Queue"=w181) -> ("Error Out"=w182:errorcluster)  [unwired: 6 in]
        }
        frame "Compute Pseudo-Phase Lifetime Plot" {
          # "\"Compute Pseudo-Phase Lifetime Plot\""
          n72 = call "Show Animated Busy Icon with Message and Abort Button.vi"("Message"="Computing Phase Lifetime Plot...", "Target VI reference"=w196) -> ("Error Out"=w200:errorcluster)  [unwired: 17 in]
          n73 = call "Compute Gated Phase Lifetime Plot Wrapper.vi"("Compute Delta Tau"=w195, "error in (no error)"=w200, "VI in"=w196) -> ("error out"=w199:errorcluster)  [unwired: 8 in]
          n74 = call "Hide Animated Busy Icon with Message and Abort Button.vi"("Target VI reference"=w196, "Error In"=w199) -> ("Error Out"=w194:errorcluster)  [unwired: 17 in]
        }
        frame "Export Parameters to Clipboard" {
          # "\"Export Parameters to Clipboard\""
          n75 = call "Show Animated Busy Icon.vi"() -> ("Error Out"=w206:errorcluster)  [unwired: 9 in]
          n76 = call "Export Parameters to Clipboard Wrapper.vi"("error in (no error)"=w206) -> ("error out"=w205:errorcluster)  [unwired: 10 in]
          n77 = call "Hide Animated Busy Icon.vi"("Error In"=w205) -> ("Error Out"=w203:errorcluster)  [unwired: 8 in]
        }
        frame "Compute alpha(beta) Plot" {
          # "\"Compute alpha(beta) Plot\""
          n78 = call "Show Animated Busy Icon with Message and Abort Button.vi"("Message"="Computing Alpha(beta) Plot...", "Target VI reference"=w211) -> ("Error Out"=w216:errorcluster)  [unwired: 17 in]
          n79 = call "Compute alpha(beta) Plot Wrapper.vi"("error in (no error)"=w216, "VI in"=w211) -> ("error out"=w215:errorcluster, "Max Tau"=→"Max Tau":dbl[unit], "Min Tau"=→"Min Tau":dbl[unit])  [unwired: 7 in]
          n80 = call "Hide Animated Busy Icon with Message and Abort Button.vi"("Error In"=w215) -> ("Error Out"=w209:errorcluster)  [unwired: 18 in]
        }
        frame "Find Pseudo UC Intersections" {
          # "\"Find Pseudo UC Intersections\""
          n81 = call "Show Animated Busy Icon with Message.vi"("Message"="Computing UC Intersections...", "Target VI reference"=w235) -> ("Error Out"=w238:errorcluster)  [unwired: 9 in]
          n82 = call "Compute f(tau) & Zeros Wrapper.vi"("VI in"=w235, "error in (no error)"=w238) -> ("Numerical Solution 1"=w223:dbl[unit], "Numerical Solution 2"=w222:dbl[unit], "Analytical Solution 1"=w220:dbl[unit], "Analytical Solution 2"=w232:dbl[unit], "error out"=w237:errorcluster)  [unwired: 9 in]
          n83 = Not A Number/Path/Refnum?(number/path/refnum=w232) -> (NaN/Path/Refnum?=w233:bool)
          n84 = Not A Number/Path/Refnum?(number/path/refnum=w220) -> (NaN/Path/Refnum?=w231:bool)
          n85 = Not(x=w233) -> (.not. x?=w229:bool)
          n86 = call "Show Animated Busy Icon with Message and Abort Button.vi"("Error In"=w237) -> ("Error Out"=w219:errorcluster)  [unwired: 18 in]
          n87 = Not(x=w231) -> (.not. x?=w230:bool)
          n88 = Or(x=w230, y=w229) -> (x .or. y?=w228:bool)
          n89 = Not A Number/Path/Refnum?(number/path/refnum=w222) -> (NaN/Path/Refnum?=w227:bool)
          n90 = property on="Analytical Solutions" class="Clust (strict)"("Visible"=w228) -> ()  [unwired: 2 in, 2 out]
          n91 = property on="Solution 2" class="DigNum (strict)"("Value"=w232, "Visible"=w229) -> ()  [unwired: 2 in, 2 out]
          n92 = Not A Number/Path/Refnum?(number/path/refnum=w223) -> (NaN/Path/Refnum?=w226:bool)
          n93 = property on="Solution 1" class="DigNum (strict)"("Value"=w220, "Visible"=w230) -> ()  [unwired: 2 in, 2 out]
          n94 = Not(x=w227) -> (.not. x?=w221:bool)
          n95 = Not(x=w226) -> (.not. x?=w225:bool)
          n96 = Or(x=w225, y=w221) -> (x .or. y?=w224:bool)
          n97 = property on="Solution 1" class="DigNum (strict)"("Value"=w223, "Visible"=w225) -> ()  [unwired: 2 in, 2 out]
          n98 = property on="Solution 2" class="DigNum (strict)"("Value"=w222, "Visible"=w221) -> ()  [unwired: 2 in, 2 out]
          n99 = property on="Numerical Solution" class="Clust (strict)"("Visible"=w224) -> ()  [unwired: 2 in, 2 out]
        }
        frame "XY Graph Special Event" {
          # "\"XY Graph Special Event\""
          n100 = Variant To Data(Variant=w244) -> (data=w245:T26, error out=w246:errorcluster)  [unwired: 2 in]
          n101 = call "XY Graph Special Event Handler Wrapper.vi"("Error In"=w246, "XY Graph Event"=w245) -> ("Error Out"=w242:errorcluster, "Message"=w243:string)  [unwired: 8 in]
          n102 = call "Send Message to Notebook.vi"("Notebook Queue"=w240, "Message"=w243, "Error In"=w242) -> ("Error Out"=w241:errorcluster)  [unwired: 16 in]
        }
        frame "Update Graph Plots Info" {
          # "\"Update Graph Plots Info\""
          n103 = call "XY Graph Get Plots Metadata.vi"("XYGraph Ref"=w252) -> ("Plots Metadata"=w251:variant[])  [unwired: 7 in, 3 out]
          n104 = Variant To Data(type=T4[] [] ("Array"), Variant=w251) -> (data=→"Phasor Graph Plots Metadata":T4[])  [unwired: 1 in, 1 out]
        }
        frame "Fit to Circle" {
          # "\"Fit to Circle\""
          n105 = Variant To Data(Variant=w264) -> (data=w263:T29, error out=w262:errorcluster)  [unwired: 2 in]
          n106 = call "Fit Plot to Circle.vi"("Full Circle Plot"=FALSE, "Error In"=w262, "Circle Fit Plot Information"=w263) -> ("Error Out"=w260:errorcluster, "Result String"=w258:string)  [unwired: 6 in, 1 out]
          n107 = call "Result Style.vi"() -> ("Default Text Formatting"=w257:T30)
          n108 = call "Send Message to Notebook.vi"("Notebook Queue"=w261, "Message"=w258, "Error In"=w260, "Text Formatting"=w257) -> ("Error Out"=w259:errorcluster)  [unwired: 15 in]
        }
        frame "Quit" {
          w271 = TRUE
          # "\"Quit\""
          n109 = call "Send Start-Stop Message.vi"("Start(T)/Stop(F)"=FALSE, "Version number"=w274, "Software Name"=w268, "Notebook Queue"=w272) -> ("Error Out"=w269:errorcluster)  [unwired: 7 in]
          n110 = call "Delete Notebook Backup on Quit.vi"("Error In"=w269, "Main VI Name"=w268) -> ("Error Out"=w267:errorcluster)  [unwired: 9 in]
          n111 = call "Phasor Explorer Save-Load Settings.vi"("Load(F)/Save (T)"=w271, "Error In"=w267) -> ("Error Out"=w270:errorcluster)  [unwired: 8 in, 1 out]
        }
      }
      n112 = Empty Array?(array=w64) -> (empty?=w63:bool)
      n113 = global write "Phasor_Abort Parallel Computation.vi" "Abort Parallel Computation"(w47) -> ()
      n114 = call "Send Error to Notebook.vi"("error in (no error)"=w54, "State Machine Case Error Source"=w51, "Notebook Q"=w53) -> ()  [unwired: 8 in, 1 out]
    }
  }
  n115 = while {
    tunnel: w32 -> [w282]
    tunnel: w17 -> [w280]
    tunnel: w15 -> [w279]
    shift-right: [w278] -> w6
    shift-left: _ -> [w277]
    stop <- w281 stop-if-true
    # "Event Loop"
    n116 = event shown="[2] \"Phasor Graph\": Cursor Move" {
      selector: w280 -> [_ _ _ _ w338 w346 w350 w358 w362 w370 _ w377 w385 w389 w397 w401 w409 _ _]
      dyn-events: [_ _ _ _ w336 w345 w348 w357 w360 w369 _ w375 w384 w387 w396 w399 w408 _ _] -> _
      timeout: _ -> [_ _ _ _ _ _ _ _ _ _ _ _ _ _ _ _ _ _ _]
      tunnel: [_ _ _ _ _ _ _ _ _ _ _ _ _ _ _ _ _ w414 w458] -> w281
      tunnel: w282 -> [_ w292 w328 w334 _ _ _ _ _ _ _ _ _ _ _ _ _ w410 w460]
      tunnel: w279 -> [_ _ _ _ _ _ _ _ _ _ _ _ _ _ _ _ _ w413 w459]
      tunnel: [w284 w290 w316 w329 w335 w341 w347 w353 w359 w365 w371 w374 w380 w386 w392 w398 w404 w412 w461] -> w278
      tunnel: w277 -> [w284 w290 w316 w329 w335 w341 w347 w353 w359 w365 w371 w374 w380 w386 w392 w398 w404 w411 w461]
      event "Abort": Value Change {
        n117 = event-data() -> ()  [unwired: 1 in, 1 out]
        n118 = global write "Phasor_Abort Parallel Computation.vi" "Abort Parallel Computation"("Abort") -> ()
        n119 = property on="Message" class="Str"() -> ("Value"=w287:string)  [unwired: 2 in, 2 out]
        n120 = Concatenate Strings(w287, ": Aborting operation, please wait..." ("string")) -> (w285:string)
        n121 = property on="Message" class="Str"("Value"=w285) -> ()  [unwired: 2 in, 2 out]
      }
      event "Phasor Graph", "Sum of Gates Graph", "Decay & Gates Graph", "f(tau) Graph", "a(b) Graph", "Pseudo-Phase Lifetime Graph": Shortcut Menu Selection (User) {
        n122 = event-data() -> ("ItemTag"=w291:string, "CtlRef"=w296:refnum<vi>, "Coords"=w295:T27, "ItemPath"=w289:string)  [unwired: 1 in]
        n123 = Bundle By Name(cluster=T26 {"Item Tag"="", "XY Graph Refnum"=refnum, "Coords"={"Horizontal"=0, "Vertical"=0}, "Item Path"=""} ("XY Graph Event"), "Item Tag"=w291, "XY Graph Refnum"=w296, "Coords"=w295, "Item Path"=w289) -> (w297:T26)
        n124 = call "Is XY Graph Special Event.vi"("XY Graph Event"=w297) -> ("XY Graph Event"=w293:T26, "Special Event"=w294:bool)  [unwired: 8 in, 1 out]
        n125 = case shown="True" w294 {
          tunnel: w293 -> [w298 w313]
          tunnel: w292 -> [w299 w315]
          tunnel: w291 -> [w300 _]
          frame False {
            n126 = case shown="\"\", Default" w300 {
              tunnel: w299 -> [_ w309]
              tunnel: w298 -> [_ w310]
              frame "", Default {
              }
              frame "Fit to Circle" {
                n127 = Unbundle(w310) -> ("XY Graph Refnum"=w305:refnum<vi>, "Coords"=w304:T27)  [unwired: 2 out]
                n128 = Bundle(cluster=T29 {"XY Graph Ref"=refnum, "Mouse Coordinates"={"X"=0.0, "Y"=0.0}, "Plot Index"=0} ("data"), "XY Graph Ref"=w305, "Mouse Coordinates"=w304, "Plot Index"=-1) -> (w303:T29)
                n129 = Bundle By Name(cluster=T22 {"ZXP Q Event"=enum."Fit to Circle", "Data"=variant} ("element"), "Data"=w303) -> (w307:T22)
                n130 = Build Array(w307) -> (w306:T22[])
                n131 = Enqueue Element(queue=w309, element=w306) -> ()  [unwired: 2 in, 3 out]
              }
            }
          }
          frame True {
            n132 = Bundle By Name(cluster=T22 {"ZXP Q Event"=enum."XY Graph Special Event", "Data"=variant} ("element"), "Data"=w313) -> (w312:T22)
            n133 = Build Array(w312) -> (w311:T22[])
            n134 = Enqueue Element(queue=w315, element=w311) -> ()  [unwired: 2 in, 3 out]
          }
        }
      }
      event "Phasor Graph": Cursor Move {
        n135 = event-data() -> ("CtlRef"=w318:refnum<vi>, "CursIdx"=w324:i32, "CursRef"=w319:refnum<vi>, "PlotIdx"=w323:i32, "PointIdx"=w322:i32, "CursLoc"=w321:cluster{"X":dbl, "Y":dbl})  [unwired: 1 in]
        n136 = Bundle By Name(cluster=T25 {"CtlRef"=refnum, "CursIdx"=0, "CursRef"=refnum, "PlotIdx"=0, "PointIdx"=0, "CursLoc"={"X"=0.0, "Y"=0.0}} ("output cluster"), "CtlRef"=w318, "CursIdx"=w324, "CursRef"=w319, "PlotIdx"=w323, "PointIdx"=w322, "CursLoc"=w321) -> (w320:T25)
        n137 = Bundle By Name(cluster=T22 {"ZXP Q Event"=enum."Update Phase & Modulus Lifetime", "Data"=variant} ("element"), "Data"=w320) -> (w326:T22)
        n138 = Build Array(w326) -> (w325:T22[])
        n139 = Enqueue Element(queue=w328, element=w325) -> ()  [unwired: 2 in, 3 out]
      }
      event "Show UC Ticks": Value Change {
        n140 = event-data() -> ("NewVal"=w332:bool)  [unwired: 1 in]
        n141 = Bundle By Name(cluster=T22 {"ZXP Q Event"=enum."Show-Hide UC Ticks", "Data"=variant} ("element"), "Data"=w332) -> (w331:T22)
        n142 = Build Array(w331) -> (w330:T22[])
        n143 = Enqueue Element(queue=w334, element=w330) -> ()  [unwired: 2 in, 3 out]
      }
      event Mouse Enter {
        n144 = event-data() -> ("CtlRef"=w339:refnum<vi>)  [unwired: 1 in]
        n145 = Unbundle By Name(w338) -> ("a(b) Graph Event Registration Refnum"=w340:refnum<event-registration>)
        n146 = call "XY Graph Tipstrip Mouse Enter.vi"("Event Registration Refnum"=w340, "XY Graph Refnum"=w339) -> ("Event Registration Refnum"=w337:refnum<event-registration>)  [unwired: 8 in, 1 out]
        n147 = Bundle By Name(cluster=w338, "a(b) Graph Event Registration Refnum"=w337) -> (w336:T23)
      }
      event Mouse Leave {
        n148 = event-data() -> ("CtlRef"=w342:refnum<vi>)  [unwired: 1 in]
        n149 = Unbundle By Name(w346) -> ("a(b) Graph Event Registration Refnum"=w344:refnum<event-registration>)
        n150 = call "XY Graph Tipstrip Mouse Leave.vi"("Event Registration Refnum"=w344, "XY Graph Refnum"=w342) -> ("Event Registration Refnum"=w343:refnum<event-registration>)  [unwired: 8 in, 1 out]
        n151 = Bundle By Name(cluster=w346, "a(b) Graph Event Registration Refnum"=w343) -> (w345:T23)
      }
      event Mouse Enter {
        n152 = event-data() -> ("CtlRef"=w351:refnum<vi>)  [unwired: 1 in]
        n153 = Unbundle By Name(w350) -> ("Decay & Gate Graph Event Registration Refnum"=w352:refnum<event-registration>)
        n154 = call "XY Graph Tipstrip Mouse Enter.vi"("Event Registration Refnum"=w352, "XY Graph Refnum"=w351) -> ("Event Registration Refnum"=w349:refnum<event-registration>)  [unwired: 8 in, 1 out]
        n155 = Bundle By Name(cluster=w350, "Decay & Gate Graph Event Registration Refnum"=w349) -> (w348:T23)
      }
      event Mouse Leave {
        n156 = event-data() -> ("CtlRef"=w354:refnum<vi>)  [unwired: 1 in]
        n157 = Unbundle By Name(w358) -> ("Decay & Gate Graph Event Registration Refnum"=w356:refnum<event-registration>)
        n158 = call "XY Graph Tipstrip Mouse Leave.vi"("Event Registration Refnum"=w356, "XY Graph Refnum"=w354) -> ("Event Registration Refnum"=w355:refnum<event-registration>)  [unwired: 8 in, 1 out]
        n159 = Bundle By Name(cluster=w358, "Decay & Gate Graph Event Registration Refnum"=w355) -> (w357:T23)
      }
      event Mouse Enter {
        n160 = event-data() -> ("CtlRef"=w363:refnum<vi>)  [unwired: 1 in]
        n161 = Unbundle By Name(w362) -> ("f(tau) Graph Event Registration Refnum"=w364:refnum<event-registration>)
        n162 = call "XY Graph Tipstrip Mouse Enter.vi"("Event Registration Refnum"=w364, "XY Graph Refnum"=w363) -> ("Event Registration Refnum"=w361:refnum<event-registration>)  [unwired: 8 in, 1 out]
        n163 = Bundle By Name(cluster=w362, "f(tau) Graph Event Registration Refnum"=w361) -> (w360:T23)
      }
      event Mouse Leave {
        n164 = event-data() -> ("CtlRef"=w366:refnum<vi>)  [unwired: 1 in]
        n165 = Unbundle By Name(w370) -> ("f(tau) Graph Event Registration Refnum"=w368:refnum<event-registration>)
        n166 = call "XY Graph Tipstrip Mouse Leave.vi"("Event Registration Refnum"=w368, "XY Graph Refnum"=w366) -> ("Event Registration Refnum"=w367:refnum<event-registration>)  [unwired: 8 in, 1 out]
        n167 = Bundle By Name(cluster=w370, "f(tau) Graph Event Registration Refnum"=w367) -> (w369:T23)
      }
      event Mouse Move {
        n168 = event-data() -> ("CtlRef"=w373:refnum<vi>, "Coords"=w372:T27)  [unwired: 1 in]
        n169 = call "XY Graph TipStrip Mouse Move.vi"("Coords"=w372, "XY Graph Refnum"=w373) -> ()  [unwired: 7 in, 3 out]
      }
      event Mouse Enter {
        n170 = event-data() -> ("CtlRef"=w378:refnum<vi>)  [unwired: 1 in]
        n171 = Unbundle By Name(w377) -> ("Phasor Graph Event Registration Refnum"=w379:refnum<event-registration>)
        n172 = call "XY Graph Tipstrip Mouse Enter.vi"("Event Registration Refnum"=w379, "XY Graph Refnum"=w378) -> ("Event Registration Refnum"=w376:refnum<event-registration>)  [unwired: 8 in, 1 out]
        n173 = Bundle By Name(cluster=w377, "Phasor Graph Event Registration Refnum"=w376) -> (w375:T23)
      }
      event Mouse Leave {
        n174 = event-data() -> ("CtlRef"=w381:refnum<vi>)  [unwired: 1 in]
        n175 = Unbundle By Name(w385) -> ("Phasor Graph Event Registration Refnum"=w383:refnum<event-registration>)
        n176 = call "XY Graph Tipstrip Mouse Leave.vi"("Event Registration Refnum"=w383, "XY Graph Refnum"=w381) -> ("Event Registration Refnum"=w382:refnum<event-registration>)  [unwired: 8 in, 1 out]
        n177 = Bundle By Name(cluster=w385, "Phasor Graph Event Registration Refnum"=w382) -> (w384:T23)
      }
      event Mouse Enter {
        n178 = event-data() -> ("CtlRef"=w390:refnum<vi>)  [unwired: 1 in]
        n179 = Unbundle By Name(w389) -> ("Pseudo-Phase Lifetime Graph Event Registration Refnum"=w391:refnum<event-registration>)
        n180 = call "XY Graph Tipstrip Mouse Enter.vi"("Event Registration Refnum"=w391, "XY Graph Refnum"=w390) -> ("Event Registration Refnum"=w388:refnum<event-registration>)  [unwired: 8 in, 1 out]
        n181 = Bundle By Name(cluster=w389, "Pseudo-Phase Lifetime Graph Event Registration Refnum"=w388) -> (w387:T23)
      }
      event Mouse Leave {
        n182 = event-data() -> ("CtlRef"=w393:refnum<vi>)  [unwired: 1 in]
        n183 = Unbundle By Name(w397) -> ("Pseudo-Phase Lifetime Graph Event Registration Refnum"=w395:refnum<event-registration>)
        n184 = call "XY Graph Tipstrip Mouse Leave.vi"("Event Registration Refnum"=w395, "XY Graph Refnum"=w393) -> ("Event Registration Refnum"=w394:refnum<event-registration>)  [unwired: 8 in, 1 out]
        n185 = Bundle By Name(cluster=w397, "Pseudo-Phase Lifetime Graph Event Registration Refnum"=w394) -> (w396:T23)
      }
      event Mouse Enter {
        n186 = event-data() -> ("CtlRef"=w402:refnum<vi>)  [unwired: 1 in]
        n187 = Unbundle By Name(w401) -> ("Sum of Gates Graph Event Registration Refnum"=w403:refnum<event-registration>)
        n188 = call "XY Graph Tipstrip Mouse Enter.vi"("Event Registration Refnum"=w403, "XY Graph Refnum"=w402) -> ("Event Registration Refnum"=w400:refnum<event-registration>)  [unwired: 8 in, 1 out]
        n189 = Bundle By Name(cluster=w401, "Sum of Gates Graph Event Registration Refnum"=w400) -> (w399:T23)
      }
      event Mouse Leave {
        n190 = event-data() -> ("CtlRef"=w405:refnum<vi>)  [unwired: 1 in]
        n191 = Unbundle By Name(w409) -> ("Sum of Gates Graph Event Registration Refnum"=w407:refnum<event-registration>)
        n192 = call "XY Graph Tipstrip Mouse Leave.vi"("Event Registration Refnum"=w407, "XY Graph Refnum"=w405) -> ("Event Registration Refnum"=w406:refnum<event-registration>)  [unwired: 8 in, 1 out]
        n193 = Bundle By Name(cluster=w409, "Sum of Gates Graph Event Registration Refnum"=w406) -> (w408:T23)
      }
      event Menu Selection (User) {
        n194 = event-data() -> ("ItemTag"=w416:string)  [unwired: 1 in]
        n195 = case shown="\"Edit User-defined Gate\"" w416 {
          tunnel: [T22[] [] ("element") T22[] [{"ZXP Q Event"=enum."Edit User-defined Gate/IRF", "Data"=variant}] ("element") T22[] [{"ZXP Q Event"=enum."Update Phasor Graph", "Data"=variant}] ("element") T22[] [{"ZXP Q Event"=enum."Update Sum of Gates Graph", "Data"=variant}] ("element") T22[] [{"ZXP Q Event"=enum."Compute Decay &/or Gates", "Data"=variant}] ("element") T22[] [{"ZXP Q Event"=enum."Find Pseudo UC Intersections", "Data"=variant}] ("element") T22[] [{"ZXP Q Event"=enum."Compute alpha(beta) Plot", "Data"=variant}] ("element") T22[] [{"ZXP Q Event"=enum."Compute Pseudo-Phase Lifetime Plot", "Data"=variant}] ("element") T22[] [{"ZXP Q Event"=enum."Update Graph Plots Info", "Data"=variant}] ("element") _ _ _ _] -> w415
          tunnel: [_ _ _ _ _ _ _ _ _ w435 _ _ _] -> w414
          tunnel: w413 -> [_ _ _ _ _ _ _ _ _ w436 w441 _ _]
          tunnel: [w417 w419 w421 w423 w425 w427 w429 w431 w433 w438 w443 w447 w453] -> w412
          tunnel: w411 -> [w417 w419 w421 w423 w425 w427 w429 w431 w433 w438 w443 w448 w452]
          tunnel: w410 -> [_ _ _ _ _ _ _ _ _ w437 _ _ _]
          frame "", Default {
          }
          frame "Edit User-defined Gate" {
          }
          frame "Update Phasor Graph" {
          }
          frame "Update Sum of Gates Graph" {
            # "deprecated"
          }
          frame "Compute Decay &/or Gates" {
          }
          frame "Find Pseudo UC Intersections" {
            # "deprecated"
          }
          frame "Compute alpha(beta) Plot" {
            # "deprecated"
          }
          frame "Compute Pseudo-Phase Lifetime Plot" {
          }
          frame "Update Graph Plots Info" {
          }
          frame "Quit" {
            n196 = call "Phasor Explorer Quit Dialog.vi"("App name"=w436, "ZXP Queue"=w437) -> ("Quit?"=w435:bool)  [unwired: 9 in]
          }
          frame "Notebook" {
            n197 = call "Set-Get Calling VI Name.vi"("Set/Get (F)"=TRUE, "Calling VI Name"=w441) -> ("Error Out"=w440:errorcluster)  [unwired: 8 in, 1 out]
            n198 = vi-ref "Notebook.vi"() -> (w445:refnum<vi>)
            n199 = property class="VI"(reference=w445, error in=w440) -> (error out=w444:errorcluster, "Path"=w442:path)  [unwired: 1 out]
            n200 = call "Run Vi.vi"("VI Path"=w442, "error in (no error)"=w444) -> ()  [unwired: 6 in, 2 out]
          }
          frame "Settings" {
            n201 = vi-ref "Phasor Explorer Settings Window.vi"() -> (w450:refnum<vi>)
            n202 = property class="VI"(reference=w450) -> (error out=w449:errorcluster, "Path"=w446:path)  [unwired: 1 in, 1 out]
            n203 = call "Run Vi.vi"("VI Path"=w446, "error in (no error)"=w449) -> ()  [unwired: 6 in, 2 out]
            n204 = call "8a583f86-e298-41fd-bd3d-00e17bb4994f.vi"("Element"=w446, "Array in"=w448) -> ("Array out"=w447:path[])  [unwired: 9 in]
          }
          frame "About" {
            n205 = vi-ref "About Phasor Explorer.vi"() -> (w455:refnum<vi>)
            n206 = property class="VI"(reference=w455) -> (error out=w454:errorcluster, "Path"=w451:path)  [unwired: 1 in, 1 out]
            n207 = call "Run Vi.vi"("VI Path"=w451, "error in (no error)"=w454, "Start Hidden? (F)"=TRUE) -> ()  [unwired: 5 in, 2 out]
            n208 = call "1c9cba52-9257-43c1-b566-a5a99626e4a7.vi"("Element"=w451, "Array in"=w452) -> ("Array out"=w453:path[])  [unwired: 9 in]
          }
        }
        n209 = Enqueue Element(queue=w410, element=w415) -> ()  [unwired: 2 in, 3 out]
      }
      event Panel Close? {
        n210 = event-data() -> ()  [unwired: 1 in, 1 out]
        n211 = call "Phasor Explorer Quit Dialog.vi"("App name"=w459, "ZXP Queue"=w460) -> ("Quit?"=w458:bool)  [unwired: 9 in]
        n212 = event-data("Discard?"=TRUE) -> ()  [unwired: 1 in, 1 out]
      }
    }
  }
  n213 = control-ref of="Display Tabs"() -> (w5:refnum<vi>)
  n214 = property class="TabCtl (strict)"(reference=w5) -> ("Pages"=w4:refnum<vi>[])  [unwired: 1 in, 2 out]
  n215 = for {
    tunnel: w4 -> [w463] mode=indexing
    tunnel: bool[] [TRUE, FALSE, FALSE, TRUE, TRUE, FALSE, FALSE] ("Page Visible") -> [w462] mode=indexing
    n216 = property class="Page"(reference=w463, "PageVis"=w462) -> ()  [unwired: 1 in, 2 out]
  }
  n217 = case shown="\"Phasor Plot\", Default" "Display Tabs" {
    frame "Phasor Plot", Default {
    }
    frame "Sum of Gates" {
    }
    frame "UC Intersections" {
    }
    frame "Alpha vs Beta" {
    }
    frame "Pseudo Phase Lifetime" {
    }
    frame "Decay, Gate & Gated Decay" {
    }
  }
  n218 = Release Queue(queue=w33) -> (error out=w27:errorcluster)  [unwired: 2 in, 2 out]
  n219 = case shown="True" w2 {
    tunnel: w27 -> [_ w469]
    tunnel: w6 -> [_ w471]
    tunnel: w1 -> [_ w470]
    frame False {
    }
    frame True {
      n220 = property class="VI"(reference=w470, error in=w469) -> (reference out=w466:refnum<vi>, error out=w465:errorcluster, "Path"=w467:path)
      n221 = Build Array (concatenate)(w471, w467) -> (w468:path[])
      n222 = Close Reference(reference=w466, error in (no error)=w465) -> (error out=w464:errorcluster)
      n223 = call "Close & Abort VIs.vi"("Error In"=w464, "VI Paths"=w468) -> ()  [unwired: 9 in, 1 out]
    }
  }
